vi "Close_USB.vi"(8 "entrée d'erreur":errorcluster caption="entrée d'erreur (pas d'erreur)", 11 "Nom de ressource VISA":refnum<visa-resource-name>) -> (0 "sortie d'erreur":errorcluster)   [LabVIEW 2014]
uses:
  <vilib>/Instr/_visa.llb/Select Event Type.ctl
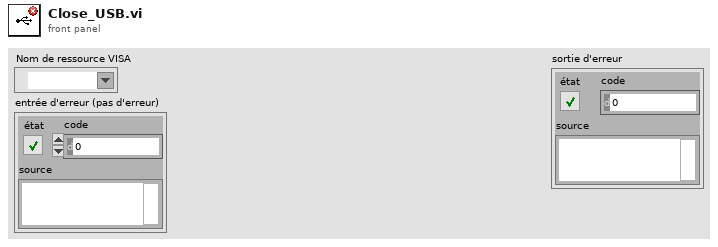
[diagram p1: front panel]
types:
  T1 = typedef "Select Event Type.ctl" = u32
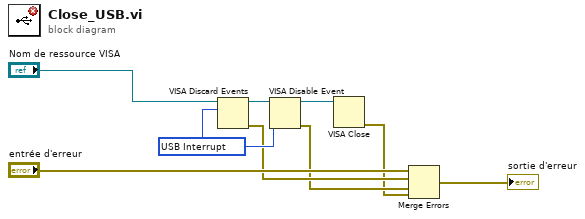
[diagram p0: block diagram]
diagram:
  w7 = T1 1073684535 items=["Service Request"=1073684491, "Trigger"=3221168138, "Clear"=1073684493, "VXI Signal"=1073684512, "VXI/VME Interrupt"=3221168161, "VXI/VME Sysfail"=1073684509, "VXI/VME Sysreset"=1073684510, "GPIB-CIC"=1073684498, "GPIB-Talk"=1073684499, "GPIB-Listen"=1073684500, "PXI Interrupt"=1073684514, "Serial Break"=1073684515, "Serial TermChar"=1073684516, "Serial CTS"=1073684521, "Serial DSR"=1073684522, "Serial DCD"=1073684524, "Serial RI"=1073684526, "Serial Character"=1073684533, "USB Interrupt"=1073684535, "All Enabled"=1073709055] ("Event Type")
  n1 = VISA Discard Events(10:w7, 11:"Nom de ressource VISA") -> (0:w4:errorcluster, 3:w9:refnum<visa-resource-name>)  [unwired: 2 in]
  n2 = VISA Disable Event(10:w7, 11:w9) -> (0:w3:errorcluster, 3:w8:refnum<visa-resource-name>)  [unwired: 2 in]
  n3 = VISA Close(VISA resource name=w8) -> (error out=w2:errorcluster)  [unwired: 1 in]
  n4 = Merge Errors("entrée d'erreur", w4, w3, w2) -> (→"sortie d'erreur":errorcluster)
